vi "KE622x -- Get Interlock State.vi"(0 "Resource In":refnum<visa-resource-name>, 1 "Check For SCPI Errors? (T)":bool=TRUE, 11 "error in (no error)":errorcluster) -> (4 "Resource Out (dupl)":refnum<visa-resource-name>, 8 "Interlock Tripped?":bool, 15 "error out":errorcluster)   [LabVIEW 2013, in "Keithly user program.lvlib"]
doc: "Used to test the Safety Interlock state. If this VI returns True, the Interlock is tripped, and thus the output is automatically disabled."
uses:
  Keithly user program.lvlib
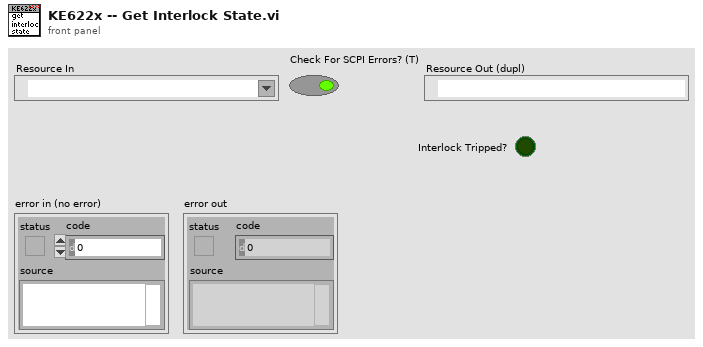
[diagram p1: front panel]
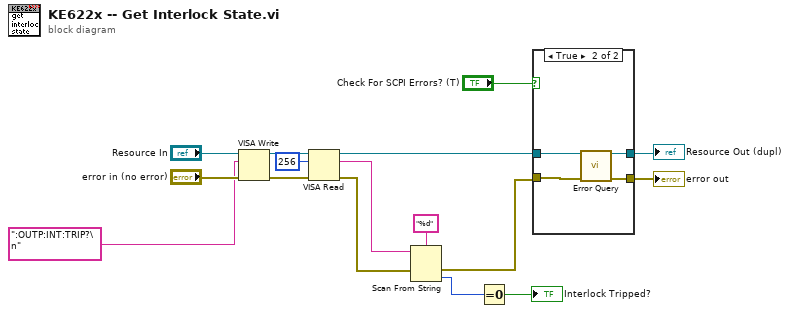
[diagram p0: block diagram]
diagram:
  n1 = VISA Write(VISA resource name="Resource In", write buffer=":OUTP:INT:TRIP?\n" ("format string"), error in (no error)="error in (no error)") -> (VISA resource name out=w10:refnum<visa-resource-name>, error out=w9:errorcluster)  [unwired: 1 out]
  n2 = VISA Read(VISA resource name=w10, byte count=u32 256, error in (no error)=w9) -> (VISA resource name out=w4:refnum<visa-resource-name>, read buffer=w3:string, error out=w7:errorcluster)  [unwired: 1 out]
  n3 = Scan From String(format string="%d", input string=w3, error in=w7) -> (error out=w5:errorcluster, output 1=w1:i32)  [unwired: 2 in, 2 out]
  n4 = Equal To 0?(x=w1) -> (x = 0?=→"Interlock Tripped?":bool)
  n5 = case shown="True" "Check For SCPI Errors? (T)" {
    tunnel: w4 -> [w18 w21]
    tunnel: w5 -> [w17 w20]
    tunnel: [w17 w19] -> w12
    tunnel: [w18 w22] -> w13
    frame False {
    }
    frame True {
      n6 = call "Error Query.vi"("VISA Resource In"=w21, "error in (no error)"=w20) -> ("VISA Resource Out (dupl)"=w22:refnum<visa-resource-name>, "error out"=w19:errorcluster)  [unwired: 10 in, 2 out]
    }
  }
  "Resource Out (dupl)" <- w13
  "error out" <- w12
